vi "Log Data Core.vi"(8 "Error In":errorcluster, 10 "Log Message":T1={"Log Action"=enum."Handle Old Files", "Variant"=variant, "Data Type"=enum."String", "Group Name"="", "Channels Names"=[]}, 11 "TDMS Log In":refnum<class "TDMS Logger.lvclass">) -> (0 "Error Out":errorcluster, 3 "TDMS Log Out":refnum<class "TDMS Logger.lvclass">)   [LabVIEW 2015, in "TDMS Logger.lvlib" / "TDMS Logger.lvclass"]
uses:
  TDMS Logger.lvclass
  _Typedefs/Log Message.ctl
  _Typedefs/Log Action.ctl
  _Typedefs/Data Type.ctl
  TDMS Logger.lvclass/TDMS Logger.ctl
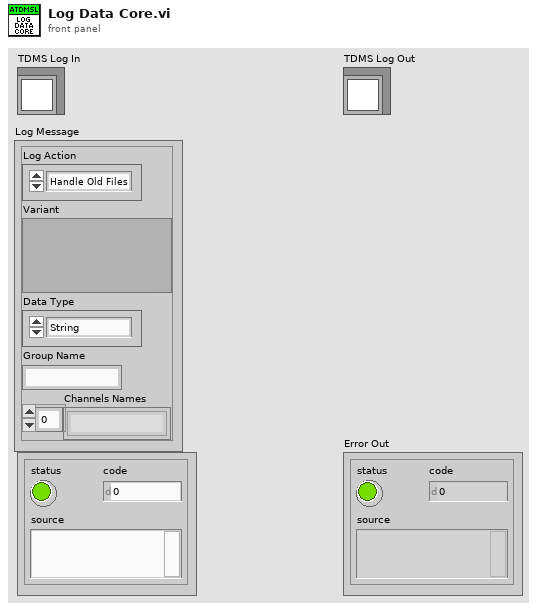
[diagram p1: front panel]
types:
  T1 = typedef "TDMS Logger.lvlib/TDMS Logger.lvclass/Log Message.ctl" = cluster{"Log Action":T2, "Variant":variant, "Data Type":T3, "Group Name":string, "Channels Names":string[]}
  T2 = typedef "TDMS Logger.lvlib/TDMS Logger.lvclass/Log Action.ctl" = enum16{"Handle Old Files", "Status Update", "Stop", "Log Data", "Initialize"}
  T3 = typedef "TDMS Logger.lvlib/TDMS Logger.lvclass/Data Type.ctl" = enum16{"I16", "I8", "String", "U16", "U8", "Waveform", "Double", "Single"}
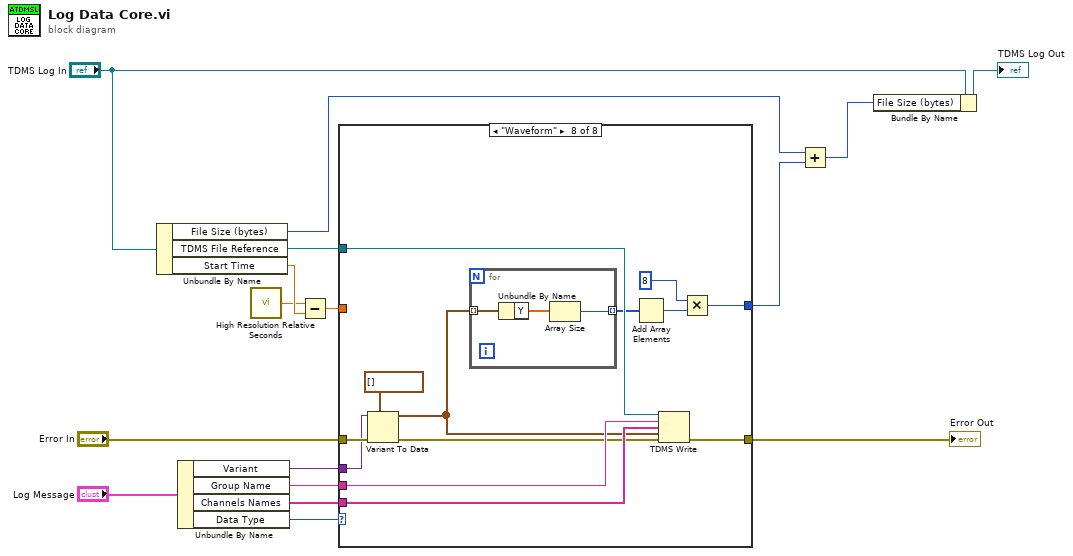
[diagram p0: block diagram]
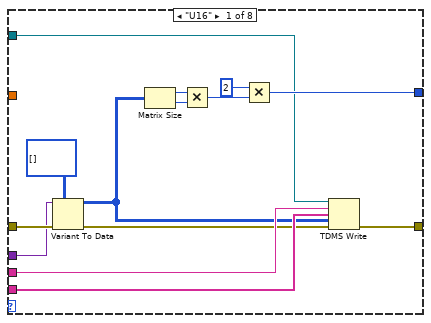
[diagram p2: hidden frame]
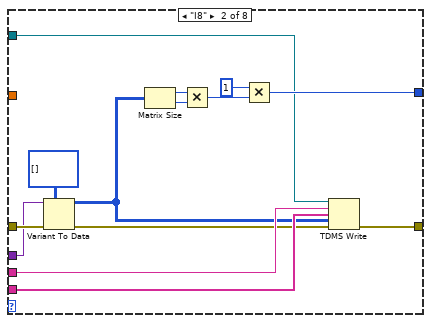
[diagram p3: hidden frame]
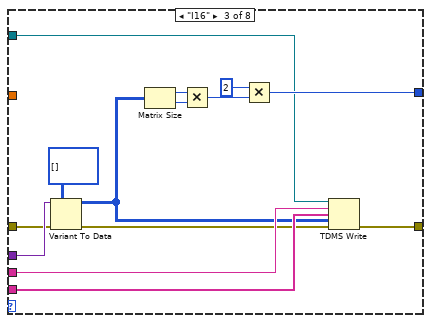
[diagram p4: hidden frame]
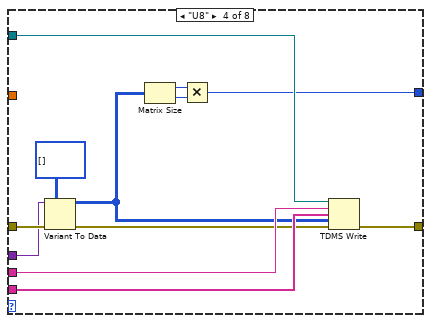
[diagram p5: hidden frame]
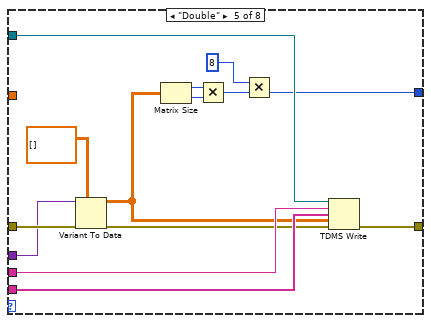
[diagram p6: hidden frame]
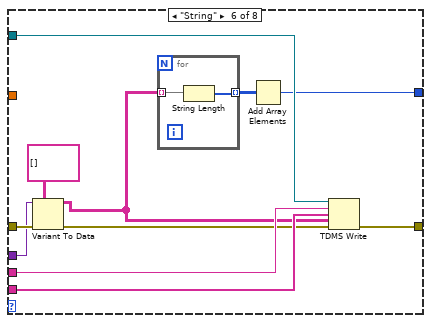
[diagram p7: hidden frame]
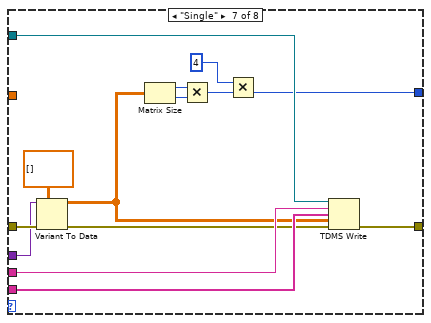
[diagram p8: hidden frame]
diagram:
  n1 = Unbundle By Name("TDMS Log In") -> ("File Size (bytes)"=w5:u64, "TDMS File Reference"=w7:refnum<k34>, "Start Time"=w3:dbl)
  n2 = Unbundle By Name("Log Message") -> ("Variant"=w4:variant, "Group Name"=w9:string, "Channels Names"=w8:string[], "Data Type"=w12:T3)
  n3 = call <vilib>:"High Resolution Relative Seconds.vi"() -> ("relative seconds"=w2:dbl)
  n4 = Subtract(x=w2, y=w3) -> (x-y=w1:dbl)
  n5 = case shown="\"Waveform\"" w12 {
    tunnel: "Error In" -> [w21 w35 w46 w63 w75 w89 w102 w116]
    tunnel: [w26 w44 w58 w64 w77 w90 w104 w120] -> w10
    tunnel: w9 -> [w25 w43 w57 w68 w82 w95 w109 w124]
    tunnel: w8 -> [w24 w42 w56 w67 w81 w94 w108 w123]
    tunnel: w7 -> [w23 w41 w55 w66 w80 w93 w107 w122]
    tunnel: [w22 w40 w54 w65 w79 w92 w106 w121] -> w6
    tunnel: w4 -> [w19 w31 w47 w59 w74 w85 w101 w112]
    tunnel: w1 -> [_ _ _ _ _ _ _ _]
    frame "U16" {
      n6 = Variant To Data(error in=w21, type=u16[][] [] ("element"), Variant=w19) -> (data=w17:u16[][], error out=w20:errorcluster)
      n7 = Matrix Size(0:w17) -> (1:w28:i32, 2:w29:i32)
      n8 = Multiply(x=w28, y=w29) -> (x*y=w27:i32)
      n9 = Multiply(x=2, y=w27) -> (x*y=w26:i32)
      n10 = TDMS Write(0:w23, 5:w25, 7:w24, 9:w17, 11:w20) -> (15:w22:errorcluster)  [unwired: 1 in, 3 out]
    }
    frame "I8" {
      n11 = Variant To Data(error in=w35, type=i8[][] [] ("element"), Variant=w31) -> (data=w32:i8[][], error out=w34:errorcluster)
      n12 = Matrix Size(0:w32) -> (1:w37:i32, 2:w38:i32)
      n13 = Multiply(x=w37, y=w38) -> (x*y=w36:i32)
      n14 = Multiply(x=1, y=w36) -> (x*y=w44:i32)
      n15 = TDMS Write(0:w41, 5:w43, 7:w42, 9:w32, 11:w34) -> (15:w40:errorcluster)  [unwired: 1 in, 3 out]
    }
    frame "I16" {
      n16 = Variant To Data(error in=w46, type=i16[][] [] ("element"), Variant=w47) -> (data=w49:i16[][], error out=w45:errorcluster)
      n17 = Matrix Size(0:w49) -> (1:w51:i32, 2:w52:i32)
      n18 = Multiply(x=w51, y=w52) -> (x*y=w50:i32)
      n19 = Multiply(x=2, y=w50) -> (x*y=w58:i32)
      n20 = TDMS Write(0:w55, 5:w57, 7:w56, 9:w49, 11:w45) -> (15:w54:errorcluster)  [unwired: 1 in, 3 out]
    }
    frame "U8" {
      n21 = Variant To Data(error in=w63, type=u8[][] [] ("element"), Variant=w59) -> (data=w60:u8[][], error out=w62:errorcluster)
      n22 = Matrix Size(0:w60) -> (1:w69:i32, 2:w70:i32)
      n23 = Multiply(x=w69, y=w70) -> (x*y=w64:i32)
      n24 = TDMS Write(0:w66, 5:w68, 7:w67, 9:w60, 11:w62) -> (15:w65:errorcluster)  [unwired: 1 in, 3 out]
    }
    frame "Double" {
      n25 = Variant To Data(error in=w75, type=dbl[][] [], Variant=w74) -> (data=w71:dbl[][], error out=w73:errorcluster)
      n26 = Matrix Size(0:w71) -> (1:w83:i32, 2:w84:i32)
      n27 = Multiply(x=w83, y=w84) -> (x*y=w78:i32)
      n28 = Multiply(x=8, y=w78) -> (x*y=w77:i32)
      n29 = TDMS Write(0:w80, 5:w82, 7:w81, 9:w71, 11:w73) -> (15:w79:errorcluster)  [unwired: 1 in, 3 out]
    }
    frame "String" {
      n30 = Variant To Data(error in=w89, type=string[][] [] ("element"), Variant=w85) -> (data=w86:string[][], error out=w88:errorcluster)
      n31 = for {
        tunnel: w86 -> [w97] mode=indexing
        tunnel: [w96] -> w91 mode=indexing
        n32 = String Length(string=w97) -> (length=w96:i32[])
      }
      n33 = Add Array Elements(numeric array=w91) -> (sum=w90:i32)
      n34 = TDMS Write(0:w93, 5:w95, 7:w94, 9:w86, 11:w88) -> (15:w92:errorcluster)  [unwired: 1 in, 3 out]
    }
    frame "Single" {
      n35 = Variant To Data(error in=w102, type=sgl[][] [] ("element"), Variant=w101) -> (data=w98:sgl[][], error out=w99:errorcluster)
      n36 = Matrix Size(0:w98) -> (1:w110:i32, 2:w111:i32)
      n37 = Multiply(x=w110, y=w111) -> (x*y=w105:i32)
      n38 = Multiply(x=4, y=w105) -> (x*y=w104:i32)
      n39 = TDMS Write(0:w107, 5:w109, 7:w108, 9:w98, 11:w99) -> (15:w106:errorcluster)  [unwired: 1 in, 3 out]
    }
    frame "Waveform" {
      n40 = Variant To Data(error in=w116, type=waveform(dbl)[] [] ("element"), Variant=w112) -> (data=w113:waveform(dbl)[], error out=w115:errorcluster)
      n41 = for {
        tunnel: w113 -> [w127] mode=indexing
        tunnel: [w125] -> w117 mode=indexing
        n42 = Unbundle By Name(w127) -> ("Y"=w126:dbl[])
        n43 = Array Size(array=w126) -> (size(s)=w125:i32)
      }
      n44 = Add Array Elements(numeric array=w117) -> (sum=w118:i32)
      n45 = TDMS Write(0:w122, 5:w124, 7:w123, 9:w113, 11:w115) -> (15:w121:errorcluster)  [unwired: 1 in, 3 out]
      n46 = Multiply(x=8, y=w118) -> (x*y=w120:i32)
    }
  }
  "Error Out" <- w6
  n47 = Add(x=w5, y=w10) -> (x+y=w13:u64)
  n48 = Bundle By Name(cluster="TDMS Log In", "File Size (bytes)"=w13) -> (→"TDMS Log Out":refnum<class "TDMS Logger.lvclass">)
